vi "PP_Raw_data_Av_Blocks.vi"() -> ()   [LabVIEW 2022 SP3]
uses:
  Globals/Meas_global.vi
  Controls/Setup.ctl
  Gen Trav/Multi_Run_Status.ctl
  Controls/File_Selector_Type.ctl
  Controls/Save_Data.ctl
panel:
  in  "No dialogs":bool
  in  "Previous Choice":path
  in  "Select Plug Ins":bool
  in  "Search String":string
  in  "Boolean":bool
  in  "Pause Mode":enum16{"Continuous Running", "After Each File"}(ring)
  in  "At Dialog Prompt Post Process":T1
  out "Files Processed":i32(slide) scale=0.0..55.0
  in  "stop":bool
  in  "File":T2=enum."Save Data"
  out "Files To Process":path[](array[path])
  in  "Post processed Results folder":path
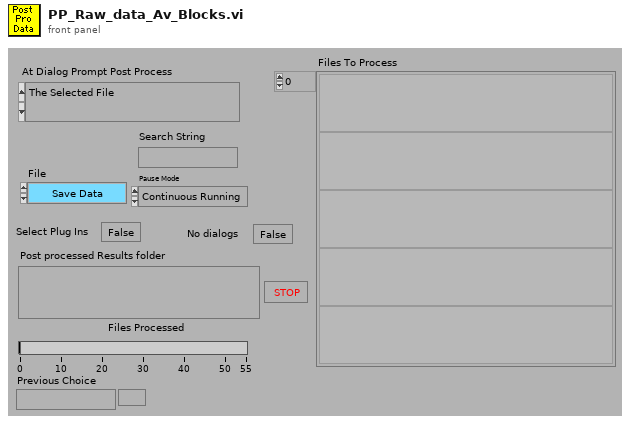
[diagram p1: front panel]
types:
  T1 = typedef "File_Selector_Type.ctl" = enum16{"The Selected File", "The Selected Folder", "Files containing the search string in the selected folder", "All files listed in selected file"}
  T2 = typedef "Save_Data.ctl" = enum16{"Save No Data", "Save Data"}
  T3 = typedef "Setup.ctl" = enum16{"Run Program", "Show Setup", "Save Current Setup", "Setup Front Panel"}
  T4 = typedef "Multi_Run_Status.ctl" = enum16{"Continue", "Continue with Error", "Jump to Next Point", "Jump to Next Row", "Jump To Fall Back", "Terminate Run"}
  T5 = enum32{"existing file", "new file", "new or existing file", "existing dir", "new dir", "new or existing dir", "existing file (use LLBs)", "new file (use LLBs)", "new or existing file (use LLBs)", "new or existing file or directory (use LLBs)"}
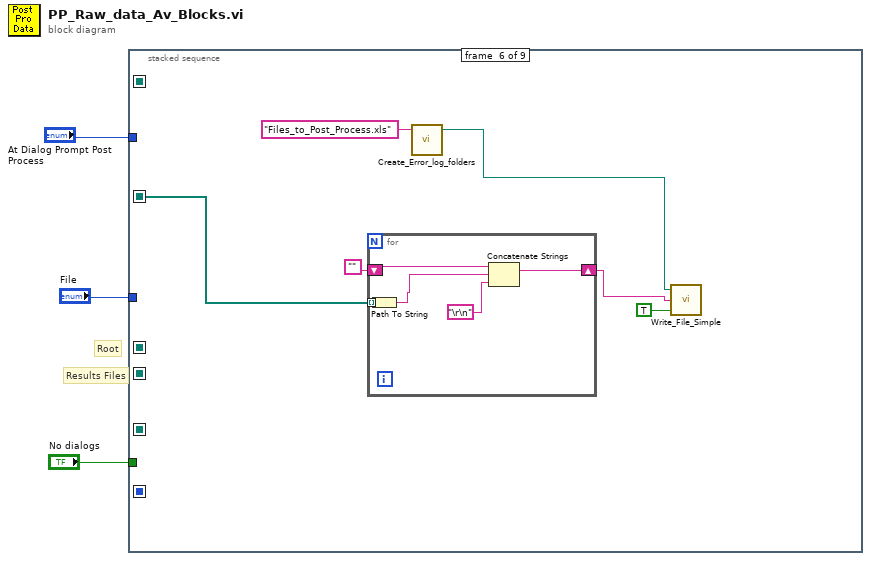
[diagram p0: block diagram]
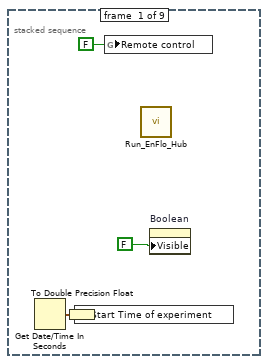
[diagram p2: hidden frame]
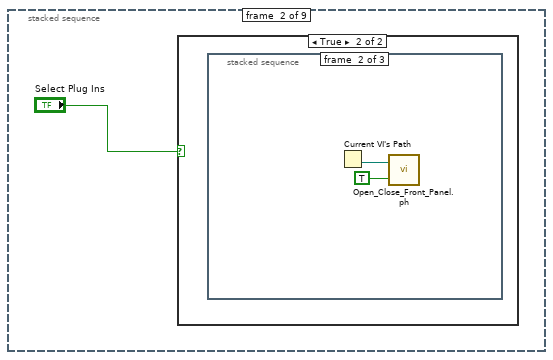
[diagram p3: hidden frame]
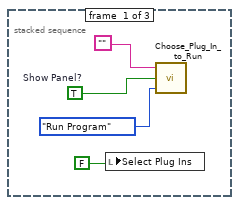
[diagram p5: hidden frame]
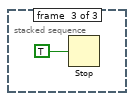
[diagram p6: hidden frame]
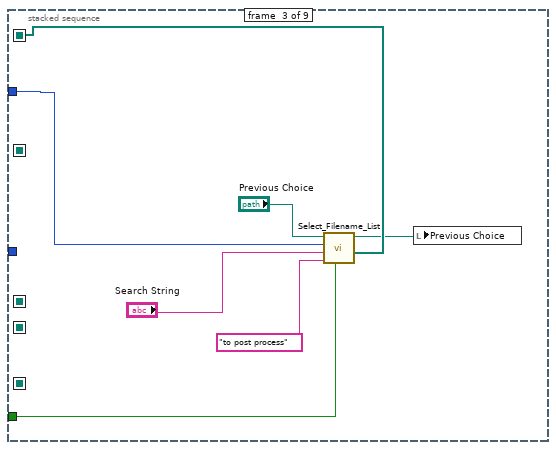
[diagram p7: hidden frame]
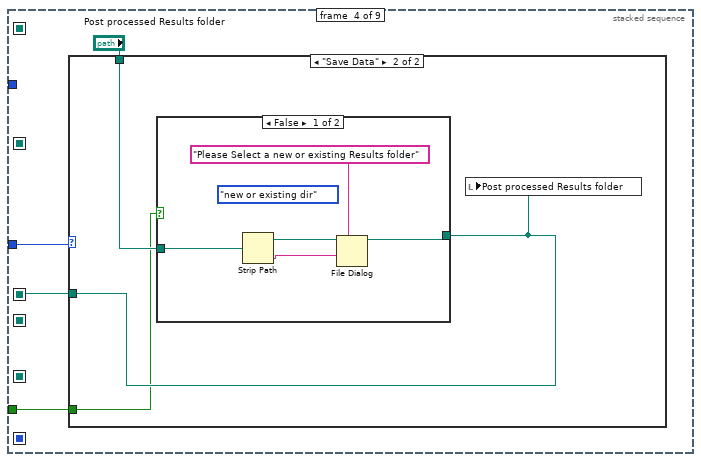
[diagram p8: hidden frame]
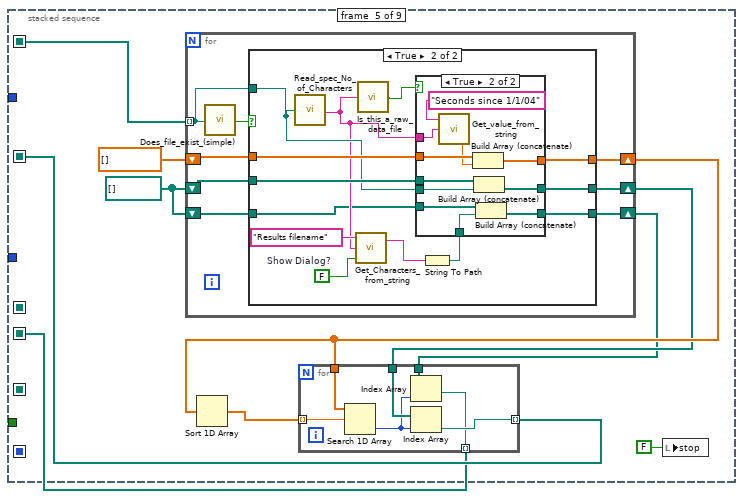
[diagram p11: hidden frame]
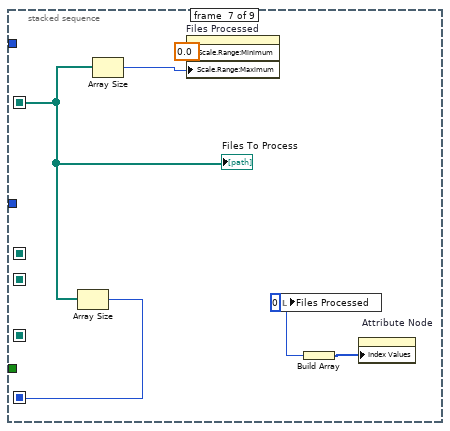
[diagram p14: hidden frame]
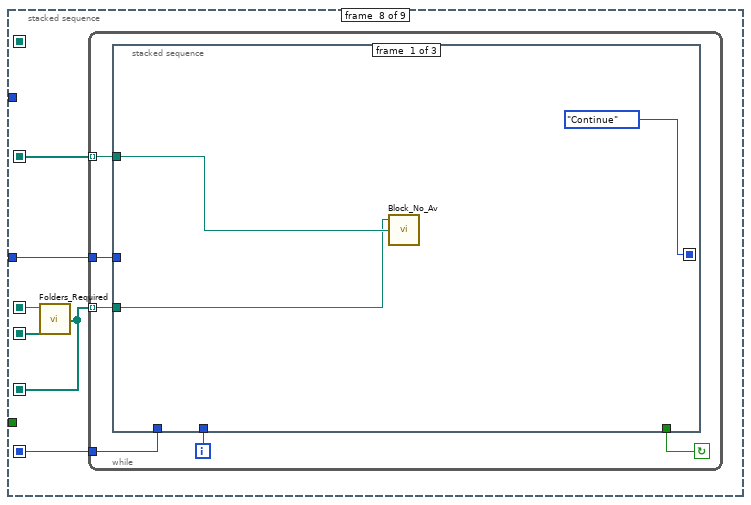
[diagram p15: hidden frame]
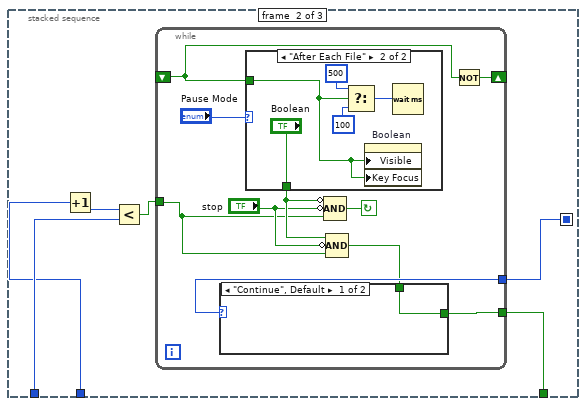
[diagram p16: hidden frame]
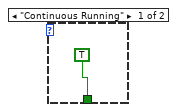
[diagram p17: hidden frame]
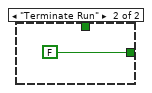
[diagram p18: hidden frame]
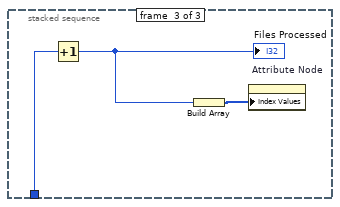
[diagram p19: hidden frame]
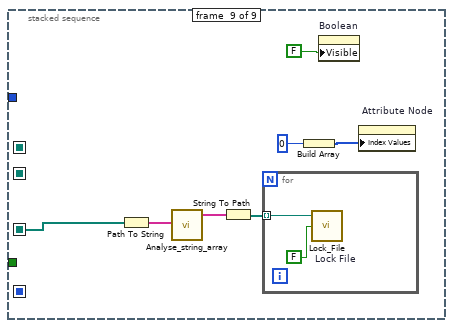
[diagram p20: hidden frame]
diagram:
  # "Root"
  # "Results Files"
  n1 = stacked-sequence {
    seq-local: [_ _ _ _ w42 _ _ _ _] -> [_ _ _ _ _ w96 w103 w114 _]
    seq-local: [_ _ _ _ _ _ w108 _ _] -> [_ _ _ _ _ _ _ w112 _]
    seq-local: [_ _ w21 _ _ _ _ _ _] -> [_ _ _ _ w40 _ _ _ _]
    seq-local: [_ _ _ w25 _ _ _ _ _] -> [_ _ _ _ _ _ _ w111 _]
    seq-local: [_ _ _ _ w37 _ _ _ _] -> [_ _ _ _ _ _ _ w110 _]
    seq-local: [_ _ _ _ _ _ _ w109 _] -> [_ _ _ _ _ _ _ _ w152]
    tunnel: "File" -> [_ _ _ w26 _ _ _ w113 _]
    tunnel: "At Dialog Prompt Post Process" -> [_ _ w22 _ _ _ _ _ _]
    tunnel: "No dialogs" -> [_ _ w16 w23 _ _ _ _ _]
    frame #0 {
      n2 = Get Date/Time In Seconds() -> (seconds since 1Jan1904=w4:timestamp)
      n3 = To Double Precision Float(number=w4) -> (double precision float=w5:dbl)
      n4 = global write "Meas_global.vi" "Start Time of experiment"(w5) -> ()
      n5 = global write "Meas_global.vi" "Remote control"(FALSE ("Remote control")) -> ()
      n6 = call "Run_EnFlo_Hub.vi"() -> ()  [unwired: 1 in, 7 out]
      n7 = property on="Boolean" class="Bool"("Visible"=FALSE ("Write Attribute")) -> ()  [unwired: 2 in, 2 out]
    }
    frame #1 {
      n8 = case shown="True" "Select Plug Ins" {
        frame False {
        }
        frame True {
          n9 = stacked-sequence {
            frame #0 {
              w12 = TRUE  # Show Panel?
              n10 = local write "Select Plug Ins"(FALSE ("Select Local ADAM Channels")) -> ()
              n11 = call "Choose_Plug_In_to_Run.vi"("setup"=Setup."Run Program", "Show Panel?"=w12, "Setup String In"="") -> ()  [unwired: 2 out]
            }
            frame #1 {
              n12 = Current VI's Path() -> (path=w14:path)
              n13 = call "Open_Close_Front_Panel.ph.vi"("openWindow (T)"=TRUE ("Front Panel Window:Open"), "VI path"=w14) -> ()  [unwired: 1 in, 1 out]
            }
            frame #2 {
              n14 = Stop(stop? (T)=TRUE) -> ()
            }
          }
        }
      }
    }
    frame #2 {
      n15 = call "Select_Filename_List.vi"("No dialogs"=w16, "File Type"="to post process", "Search String"="Search String", "At Dialog Prompt Post Process"=w22, "Previous Choice"="Previous Choice") -> ("Selected files"=w21:path[], "Choosen path"=w17:path)  [unwired: 2 out]
      n16 = local write "Previous Choice"(w17) -> ()
    }
    frame #3 {
      n17 = case shown="\"Save Data\"" w26 {
        tunnel: [w27 w30] -> w25
        tunnel: "Post processed Results folder" -> [w27 w29]
        tunnel: w23 -> [_ w28]
        frame "Save No Data" {
        }
        frame "Save Data" {
          n18 = case shown="False" w28 {
            tunnel: [w35 w36] -> w30
            tunnel: w29 -> [w33 w36]
            frame False {
              (unwired) T5."new or existing dir" ("select mode (2)")
              n19 = Strip Path(path=w33) -> (stripped path=w32:path, name=w31:string)
              n20 = File Dialog(7:"Please Select a new or existing Results folder" ("prompt"), 9:w31, 11:w32) -> (3:w35:path)  [unwired: 1 in, 6 out]
            }
            frame True {
            }
          }
          n21 = local write "Post processed Results folder"(w30) -> ()
        }
      }
    }
    frame #4 {
      w39 = path[] []
      n22 = for {
        tunnel: w40 -> [w56] mode=indexing
        shift-right: [w60] -> w46
        shift-left: dbl[] [] -> [w61]
        shift-right: [w58] -> w43
        shift-left: w39 -> [w59]
        shift-right: [w54] -> w38
        shift-left: w39 -> [w55]
        n23 = call "Does_file_exist_(simple).vi"("Pathname"=w56) -> ("exists?"=w57:bool)
        n24 = case shown="True" w57 {
          tunnel: w61 -> [w64 w77]
          tunnel: [w64 w76] -> w60
          tunnel: w59 -> [w63 w75]
          tunnel: [w63 w74] -> w58
          tunnel: w56 -> [_ w72]
          tunnel: w55 -> [w62 w67]
          tunnel: [w62 w66] -> w54
          frame False {
          }
          frame True {
            w70 = FALSE  # Show Dialog?
            n25 = call "Read_spec_No_of_Characters.vi"("Filename"=w72) -> ("character string"=w69:string)  [unwired: 1 out]
            n26 = call "Get_Characters_from_string.vi"("Show Dialog?"=w70, "Input string"=w69, "Variable name"="Results filename") -> ("Value"=w65:string)  [unwired: 1 out]
            n27 = call "Is_this_a_raw_data_file.vi"("character string"=w69) -> ("Raw Dat File?"=w73:bool)  [unwired: 2 out]
            n28 = String To Path(string=w65) -> (path=w68:path)
            n29 = case shown="True" w73 {
              tunnel: w77 -> [w80 w89]
              tunnel: [w80 w91] -> w76
              tunnel: w75 -> [w79 w87]
              tunnel: w72 -> [_ w86]
              tunnel: [w79 w85] -> w74
              tunnel: w69 -> [_ w84]
              tunnel: w68 -> [_ w83]
              tunnel: w67 -> [w78 w82]
              tunnel: [w78 w81] -> w66
              frame False {
              }
              frame True {
                n30 = call "Get_value_from_string.vi"("Input string"=w84, "Variable name"="Seconds since 1/1/04") -> ("Value"=w88:dbl)  [unwired: 1 in, 1 out]
                n31 = Build Array (concatenate)(w89, w88) -> (w91:dbl[])
                n32 = Build Array (concatenate)(w87, w86) -> (w85:path[])
                n33 = Build Array (concatenate)(w82, w83) -> (w81:path[])
              }
            }
          }
        }
      }
      n34 = Sort 1D Array(array=w46) -> (sorted array=w45:dbl[])
      n35 = for {
        tunnel: w46 -> [w53]
        tunnel: w45 -> [w52] mode=indexing
        tunnel: w43 -> [w51]
        tunnel: [w50] -> w42 mode=indexing
        tunnel: w38 -> [w48]
        tunnel: [w47] -> w37 mode=indexing
        n36 = Search 1D Array(1D array=w53, element=w52) -> (index of element=w49:i32)  [unwired: 1 out]
        n37 = Index Array(array=w48, index=w49) -> (element=w47:path)
        n38 = Index Array(array=w51, index=w49) -> (element=w50:path)
      }
      n39 = local write "stop"(FALSE ("stop")) -> ()
    }
    frame #5 {
      n40 = for {
        shift-right: [w98] -> w92
        shift-left: "" -> [w102]
        tunnel: w96 -> [w100] mode=indexing
        n41 = Path To String(path=w100) -> (string=w99:string)
        n42 = Concatenate Strings(w102, w99, "\r\n") -> (w98:string)
      }
      n43 = call "Create_Error_log_folders.vi"("Log Filename"="Files_to_Post_Process.xls") -> ("Local Log File"=w93:path)  [unwired: 5 in, 1 out]
      n44 = call "Write_File_Simple.vi"("append to file? (new file:F)"=TRUE, "character string"=w92, "file path"=w93) -> ()  [unwired: 2 out]
    }
    frame #6 {
      w104 = 0 ("Files Processed")
      n45 = Array Size(array=w103) -> (size(s)=w108:i32)
      n46 = Array Size(array=w103) -> (size(s)=w106:i32)
      n47 = property on="Files Processed" class="Slide (strict)"("Scale.Range:Minimum"=0.0 ("Write Attribute"), "Scale.Range:Maximum"=w106) -> ()  [unwired: 2 in, 2 out]
      n48 = local write "Files Processed"(w104) -> ()
      n49 = Build Array(w104) -> (w105:i32[])
      n50 = property on="Attribute Node" class="Arr (strict)"("Index Values"=w105) -> ()  [unwired: 2 in, 2 out]
      "Files To Process" <- w103
    }
    frame #7 {
      n51 = call "Folders_Required.vi"("Filenames"=w110, "New Root"=w111) -> ("Array"=w109:path[])  [unwired: 2 in]
      n52 = while {
        tunnel: w109 -> [w115] mode=indexing
        tunnel: w112 -> [w118]
        tunnel: w113 -> [w119]
        tunnel: w114 -> [w120] mode=indexing
        i -> [w117]
        stop <- w116 continue-if-true
        n53 = stacked-sequence {
          seq-local: [Multi_Run_Status."Continue" ("Status Out") _ _] -> [_ w125 _]
          tunnel: w115 -> [w121 _ _]
          tunnel: w120 -> [w122 _ _]
          tunnel: w119 -> [_ _ _]
          tunnel: w118 -> [_ w127 _]
          tunnel: w117 -> [_ w126 w149]
          tunnel: [_ w124 _] -> w116
          frame #0 {
            n54 = call "Block_No_Av.vi"("Raw data file"=w122, "Results file"=w121) -> ()  [unwired: 3 in]
          }
          frame #1 {
            n55 = Increment(x=w126) -> (x+1=w129:i32)
            n56 = Less?(x=w129, y=w127) -> (x < y?=w128:bool)
            n57 = while {
              shift-left: _ -> [w135]
              shift-right: [w136] -> _
              tunnel: [w138] -> w124
              tunnel: w125 -> [w139]
              tunnel: w128 -> [w131]
              stop <- w134 continue-if-true
              n58 = case shown="\"After Each File\"" "Pause Mode" {
                tunnel: [TRUE "Boolean"] -> w133
                tunnel: w135 -> [_ w144]
                frame "Continuous Running" {
                }
                frame "After Each File" {
                  n59 = Select(t=u32 500 ("milliseconds to wait"), s=w144, f=u32 100) -> (s? t:f=w141:u32)
                  n60 = property on="Boolean" class="Bool"("Visible"=w144, "Key Focus"=w144) -> ()  [unwired: 2 in, 2 out]
                  n61 = Wait (ms)(milliseconds to wait=w141) -> ()  [unwired: 1 out]
                }
              }
              n62 = Compound Arithmetic op=AND(invert w133, invert "stop", w131) -> (w134:bool)
              n63 = Compound Arithmetic op=AND(w133, invert "stop", w131) -> (w130:bool)
              n64 = case shown="\"Continue\", Default" w139 {
                tunnel: [w146 FALSE] -> w138
                tunnel: w130 -> [w146 _]
                frame "Continue", Default {
                }
                frame "Terminate Run" {
                }
              }
              n65 = Not(x=w135) -> (.not. x?=w136:bool)
            }
          }
          frame #2 {
            n66 = Increment(x=w149) -> (x+1=w148:i32)
            "Files Processed" <- w148
            n67 = Build Array(w148) -> (w150:i32[])
            n68 = property on="Attribute Node" class="Arr (strict)"("Index Values"=w150) -> ()  [unwired: 2 in, 2 out]
          }
        }
      }
    }
    frame #8 {
      n69 = Path To String(path=w152) -> (string=w154:string[])
      n70 = call "Analyse_string_array.vi"("String array"=w154) -> ("Unique strings"=w153:string[])  [unwired: 2 out]
      n71 = String To Path(string=w153) -> (path=w151:path[])
      n72 = for {
        tunnel: w151 -> [w158] mode=indexing
        w159 = FALSE  # Lock File
        n73 = call "Lock_File.vi"("Lock File"=w159, "path"=w158) -> ()  [unwired: 1 in, 3 out]
      }
      n74 = Build Array(0) -> (w156:i32[])
      n75 = property on="Boolean" class="Bool"("Visible"=FALSE ("Write Attribute")) -> ()  [unwired: 2 in, 2 out]
      n76 = property on="Attribute Node" class="Arr (strict)"("Index Values"=w156) -> ()  [unwired: 2 in, 2 out]
    }
  }
